vi "FMA1600A Create Custom Gas Mixture.vi"(6 "Gas Mix Number":string, 7 "Gas Type":T1, 8 "Error In":errorcluster, 9 "Custom Gas Mixture":string, 10 "Unit ID":string, 11 "VISA Refnum in":refnum<visa-resource-name>) -> (0 "Error Out":errorcluster)   [LabVIEW 2016]
uses:
  Type Definitions/FMA1600A Gas Type.ctl
  Type Definitions/FMA1600A Commands.ctl
panel:
  out "VISA Refnum out":refnum<visa-resource-name>
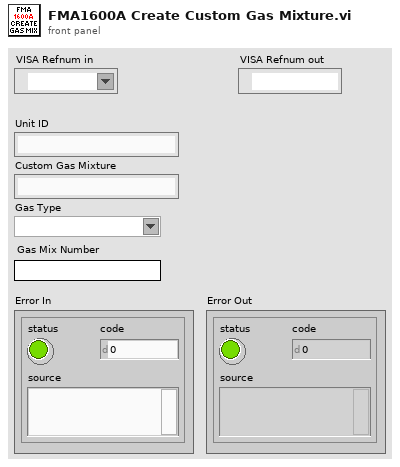
[diagram p1: front panel]
types:
  T1 = typedef "FMA1600A Gas Type.ctl" = string
  T2 = typedef "FMA1600A Commands.ctl" = string
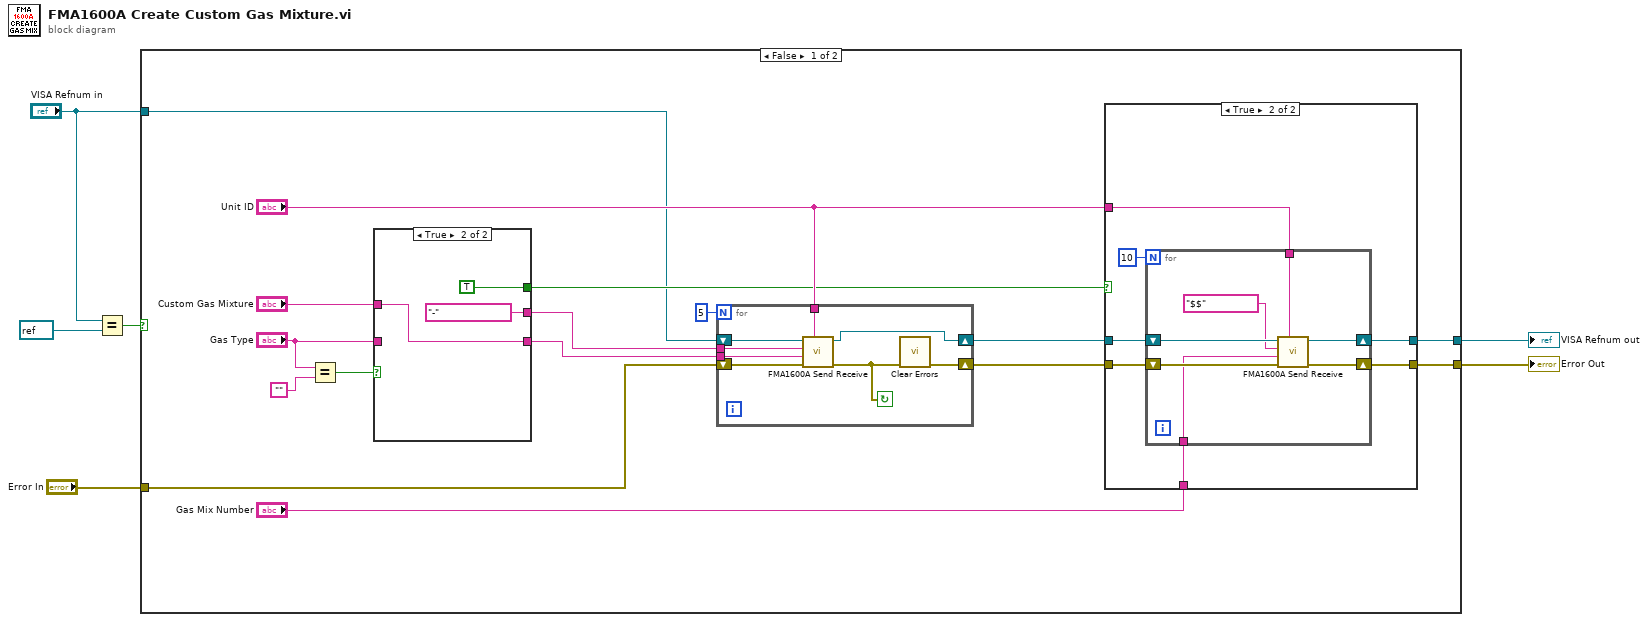
[diagram p0: block diagram]
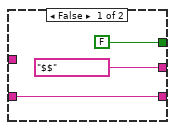
[diagram p3: hidden frame]
diagram:
  n1 = Equal?(x="VISA Refnum in", y=refnum<visa-resource-name> refnum) -> (x = y?=w4:bool)
  n2 = case shown="False" w4 {
    tunnel: "VISA Refnum in" -> [w16 w53]
    tunnel: [w15 w53] -> w6
    tunnel: [w14 w54] -> w5
    tunnel: "Error In" -> [w7 w54]
    frame False {
      n3 = Equal?(x="Gas Type", y="") -> (x = y?=w11:bool)
      n4 = case shown="True" w11 {
        tunnel: [w47 w50] -> w17
        tunnel: [T2 "$$" ("FMA1600A Commands") T2 "-" ("FMA1600A Commands")] -> w18
        tunnel: [FALSE TRUE] -> w19
        tunnel: "Custom Gas Mixture" -> [_ w50]
        tunnel: "Gas Type" -> [w47 _]
        frame False {
        }
        frame True {
        }
      }
      n5 = for {
        N: 5 -> [_]
        tunnel: "Unit ID" -> [w30]
        tunnel: w18 -> [w28]
        tunnel: w17 -> [w27]
        shift-right: [w29] -> w20
        shift-left: w16 -> [w26]
        shift-right: [w23] -> w9
        shift-left: w7 -> [w25]
        stop <- w24 continue-if-true
        n6 = call "FMA1600A Send Receive.vi"("Unit ID"=w30, "error in (no error)"=w25, "Gas Type"=w27, "FMA1600A Commands"=w28, "VISA Refnum in"=w26) -> ("error out"=w24:errorcluster, "VISA Refnum out"=w29:refnum<visa-resource-name>)  [unwired: 4 in, 1 out]
        n7 = call <vilib>:"Clear Errors.vi"("error in (no error)"=w24) -> ("error out"=w23:errorcluster)  [unwired: 5 in, 1 out]
      }
      n8 = case shown="True" w19 {
        tunnel: w9 -> [w32 w39]
        tunnel: [w32 w38] -> w14
        tunnel: w20 -> [w31 w37]
        tunnel: "Unit ID" -> [_ w36]
        tunnel: "Gas Mix Number" -> [_ w35]
        tunnel: [w31 w34] -> w15
        frame False {
        }
        frame True {
          n9 = for {
            N: 10 -> [_]
            tunnel: w36 -> [w43]
            tunnel: w35 -> [w41]
            shift-right: [w45] -> w38
            shift-left: w39 -> [w46]
            shift-right: [w40] -> w34
            shift-left: w37 -> [w44]
            n10 = call "FMA1600A Send Receive.vi"("Unit ID"=w43, "error in (no error)"=w46, "Gas Type"=w41, "FMA1600A Commands"=T2 "$$", "VISA Refnum in"=w44) -> ("error out"=w45:errorcluster, "VISA Refnum out"=w40:refnum<visa-resource-name>)  [unwired: 4 in, 1 out]
          }
        }
      }
    }
    frame True {
    }
  }
  "Error Out" <- w5
  "VISA Refnum out" <- w6
